vi "ParseArguments.vi"(8 "error in (no error)":errorcluster, 9 "Inputs":string[](array[string]), 11 "DiffVI in":refnum<class "DiffVI.lvclass">) -> (0 "error out":errorcluster, 3 "DiffVI out":refnum<class "DiffVI.lvclass">)   [LabVIEW 2015, in "DiffVI.lvclass"]
uses:
  DiffVI.lvclass
  DiffVI.lvclass/DiffVI.ctl
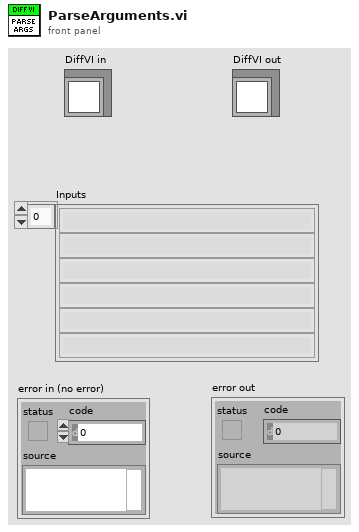
[diagram p1: front panel]
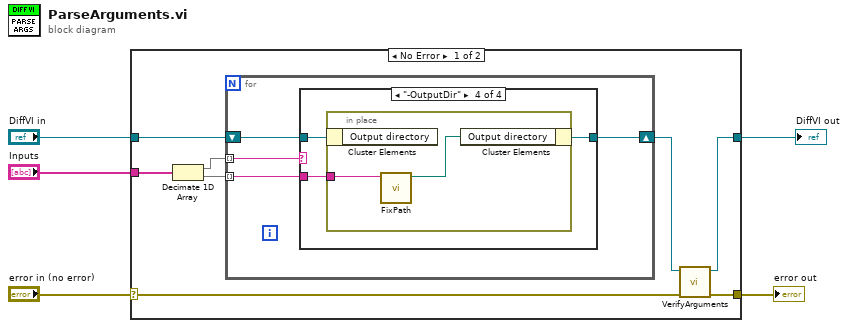
[diagram p0: block diagram]
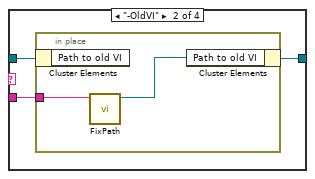
[diagram p3: hidden frame]
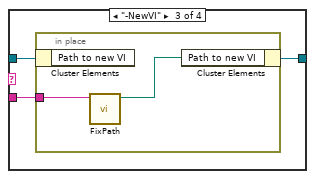
[diagram p4: hidden frame]
diagram:
  n1 = case shown="No Error" "error in (no error)" {
    selector: "error in (no error)" -> [w8 w35]
    tunnel: [w9 w35] -> w4
    tunnel: "DiffVI in" -> [w11 w34]
    tunnel: "Inputs" -> [w10 _]
    tunnel: [w6 w34] -> w1
    frame No Error {
      n2 = Decimate 1D Array(w10) -> (w12:string[], w13:string[])
      n3 = for {
        tunnel: w12 -> [w17] mode=indexing
        tunnel: w13 -> [w15] mode=indexing
        shift-right: [w14] -> w7
        shift-left: w11 -> [w16]
        n4 = case shown="\"-OutputDir\"" w17 {
          tunnel: w16 -> [w18 w21 w26 w31]
          tunnel: w15 -> [_ w20 w25 w30]
          tunnel: [w18 w19 w24 w29] -> w14
          frame Default {
          }
          frame "-OldVI" {
            n5 = in-place {
              in-place-border: w20 -> [w23]
              n6 = in-place-cluster #1(w21) -> ()  [unwired: 1 out]
              n7 = call "FixPath.vi"("path string"=w23) -> ("path"=w22:path)  [unwired: 10 in]
              n8 = in-place-cluster #1("Path to old VI"=w22) -> (w19:refnum<class "DiffVI.lvclass">)
            }
          }
          frame "-NewVI" {
            n9 = in-place {
              in-place-border: w25 -> [w28]
              n10 = in-place-cluster #2(w26) -> ()  [unwired: 1 out]
              n11 = call "FixPath.vi"("path string"=w28) -> ("path"=w27:path)  [unwired: 10 in]
              n12 = in-place-cluster #2("Path to new VI"=w27) -> (w24:refnum<class "DiffVI.lvclass">)
            }
          }
          frame "-OutputDir" {
            n13 = in-place {
              in-place-border: w30 -> [w33]
              n14 = in-place-cluster #3(w31) -> ()  [unwired: 1 out]
              n15 = call "FixPath.vi"("path string"=w33) -> ("path"=w32:path)  [unwired: 10 in]
              n16 = in-place-cluster #3("Output directory"=w32) -> (w29:refnum<class "DiffVI.lvclass">)
            }
          }
        }
      }
      n17 = call "VerifyArguments.vi"("error in (no error)"=w8, "DiffVI in"=w7) -> ("error out"=w9:errorcluster, "DiffVI out"=w6:refnum<class "DiffVI.lvclass">)  [unwired: 8 in]
    }
    frame Error {
    }
  }
  "error out" <- w4
  "DiffVI out" <- w1
